vi "DrawClockAsQTImage.vi"(1 "Clock Bounds":cluster{"Width":u32, "Height":u32}={"Width"=100, "Height"=100}, 5 "frame ID":i32=54) -> (14 "Picture":picture, 17 "Image Out (24 bits)":T3={"Width"=220, "Height"=151, "Depth"=24, "data"=array[99660 elements], "Compressed data"=[], "Color table"=[], "Duration"=0, "Options"=0, "Timestamp"=0, "ID"=1, "Reserved"=0, "Dialogs"=0} {"Dialogs" format="%.0b"})   [LabVIEW 2024]
uses:
  <userlib>/ImageProcessing/QTLIB_2595_LV86/QT_Image.ctl
  <vilib>/picture/picture.llb/imagedata.ctl
panel:
  out "new picture 2":picture
  out "image data 2":T1={"image type"=0, "image depth"=24, "image"=array[99660 elements], "mask"=[], "colors"=[], "Rectangle"={"left"=0, "top"=0, "right"=220, "bottom"=151}}
  out "image data":T2={"image type"=0, "image depth"=24, "image"=array[93090 elements], "mask"=[], "colors"=[], "Rectangle"={"left"=0, "top"=0, "right"=214, "bottom"=145}}
  out "new picture":picture
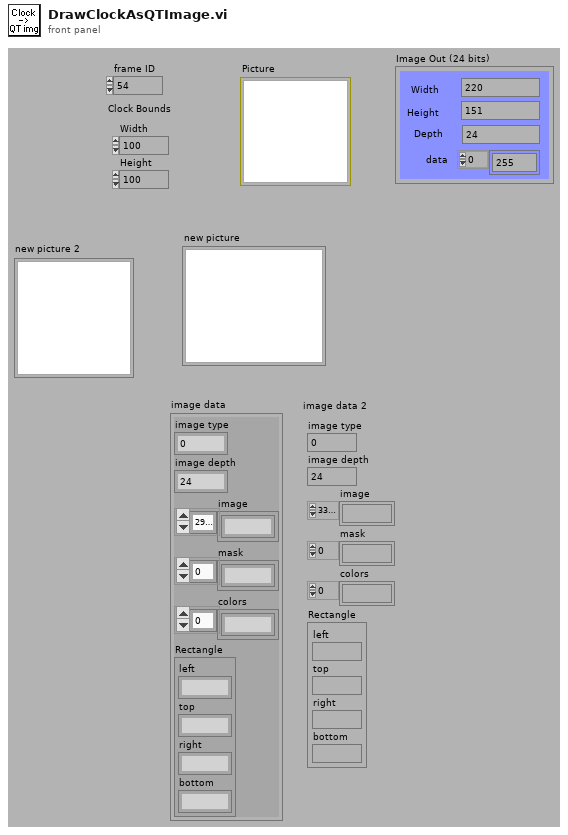
[diagram p1: front panel]
types:
  T1 = cluster{"image type":i32, "image depth":i32, "image":u8[], "mask":u8[], "colors":u32[], "Rectangle":cluster{"left":i16, "top":i16, "right":i16, "bottom":i16}}
  T2 = typedef "imagedata.ctl" = cluster{"image type":i32, "image depth":i32, "image":u8[], "mask":u8[], "colors":u32[], "Rectangle":cluster{"left":i16, "top":i16, "right":i16, "bottom":i16}}
  T3 = typedef "QT_Image.ctl" = cluster{"Width":i32, "Height":i32, "Depth":i32, "data":u8[], "Compressed data":u8[], "Color table":u32[], "Duration":i32, "Options":i32, "Timestamp":i32, "ID":i32, "Reserved":i32, "Dialogs":u32}
  T4 = cluster{"left":i16, "top":i16, "right":i16, "bottom":i16}
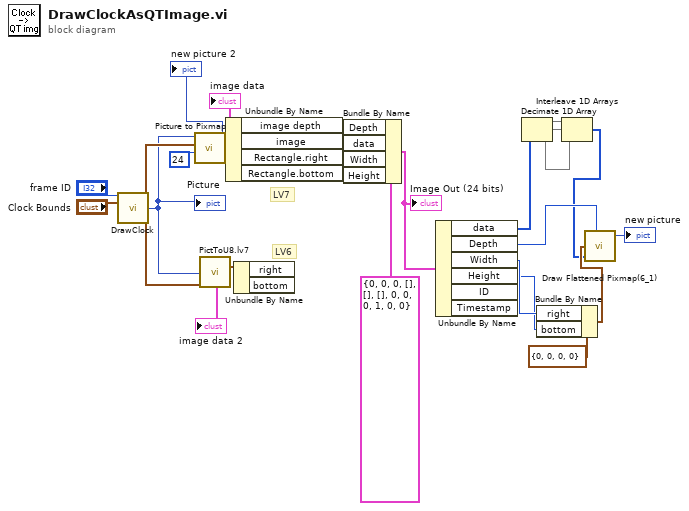
[diagram p0: block diagram]
diagram:
  # "LV6"
  # "LV7"
  n1 = call <userlib>:"DrawClock.vi"("Frame idx"="frame ID", "Draw Area Size"="Clock Bounds") -> ("Picture Draw Area Size"=w24:cluster{"Width":u32, "Height":u32}, "clock picture"=w6:picture, "Picture Rect"=w11:T4)  [unwired: 1 in, 10 out]
  "Picture" <- w6
  n2 = call <vilib>:"Picture to Pixmap.vi"("depth"=24, "rect"=w11, "picture"=w6) -> ("image data"=w5:T2, "new picture"=→"new picture 2":picture)  [unwired: 1 in, 6 out]
  "image data" <- w5
  n3 = call <userlib>:"PictToU8.lv7.vi"("picture"=w6, "Draw Area Size"=w24) -> ("image rect"=w8:T4, "image data"=→"image data 2":T1)  [unwired: 12 out]
  n4 = Unbundle By Name(w5) -> ("image depth"=w4:i32, "image"=w3:u8[], "Rectangle.right"=w2:i16, "Rectangle.bottom"=w1:i16)
  n5 = Unbundle By Name(w8) -> ()  [unwired: 2 out]
  n6 = Bundle By Name(cluster=T3 {"Width"=0, "Height"=0, "Depth"=0, "data"=[], "Compressed data"=[], "Color table"=[], "Duration"=0, "Options"=0, "Timestamp"=0, "ID"=1, "Reserved"=0, "Dialogs"=0} ("Image in"), "Depth"=w4, "data"=w3, "Width"=w2, "Height"=w1) -> (w23:T3)
  "Image Out (24 bits)" <- w23
  n7 = Unbundle By Name(w23) -> ("data"=w13:u8[], "Depth"=w17:i32, "Width"=w19:i32, "Height"=w18:i32)  [unwired: 2 out]
  n8 = Decimate 1D Array(w13) -> (w16:u8[], w15:u8[], w14:u8[])
  n9 = Bundle By Name(cluster=T4 {"left"=0, "top"=0, "right"=0, "bottom"=0} ("rect"), "right"=w19, "bottom"=w18) -> (w21:T4)
  n10 = Interleave 1D Arrays(w16, w15, w14) -> (w12:u8[])
  n11 = call <vilib>:"Draw Flattened Pixmap(6_1).vi"("bit depth(8)"=w17, "rect"=w21, "flattened pixmap data"=w12) -> ("new picture"=→"new picture":picture)  [unwired: 2 in, 4 out]
